vi "DEMO_02_READ_VOLT_S.vi"() -> ()   [LabVIEW 2018]
uses:
  <vilib>/Instr/_visa.llb/VISA Configure Serial Port (Instr).vi
panel:
  out "输出变量":dbl
  in  "打开串口":bool
  in  "通道选择":enum16{"一路", "二路", "三路"}(ring)
  in  "开闭环":u16(ring) items=["  开环", "  闭环"]
  in  "上位机控制":bool
  in  "读取数据":bool
  in  "VISA资源名称":refnum<visa-resource-name>="COM1"
  in  "波特率":u32(ring)=9600 items=["75"=75, "110"=110, "134"=134, "150"=150, "300"=300, "600"=600, "1200"=1200, "1800"=1800, "2400"=2400, "4800"=4800, "7200"=7200, "9600"=9600, "14400"=14400, "19200"=19200, "28800"=28800, "38400"=38400, "56000"=56000, "57600"=57600, "115200"=115200, "128000"=128000, "230400"=230400]
  in  "奇偶":enum16{"None", "Odd", "Even", "Mark", "Space"}(ring) caption="校验"
  # "发送数据以及读取开闭环数据"
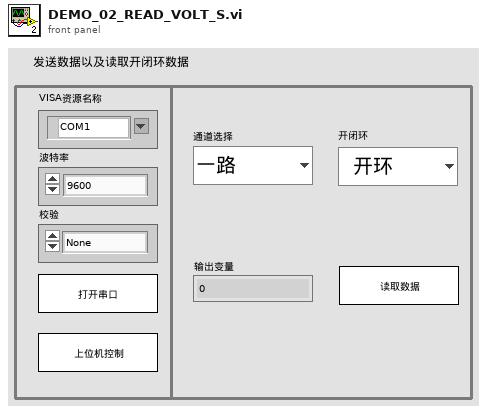
[diagram p1: front panel]
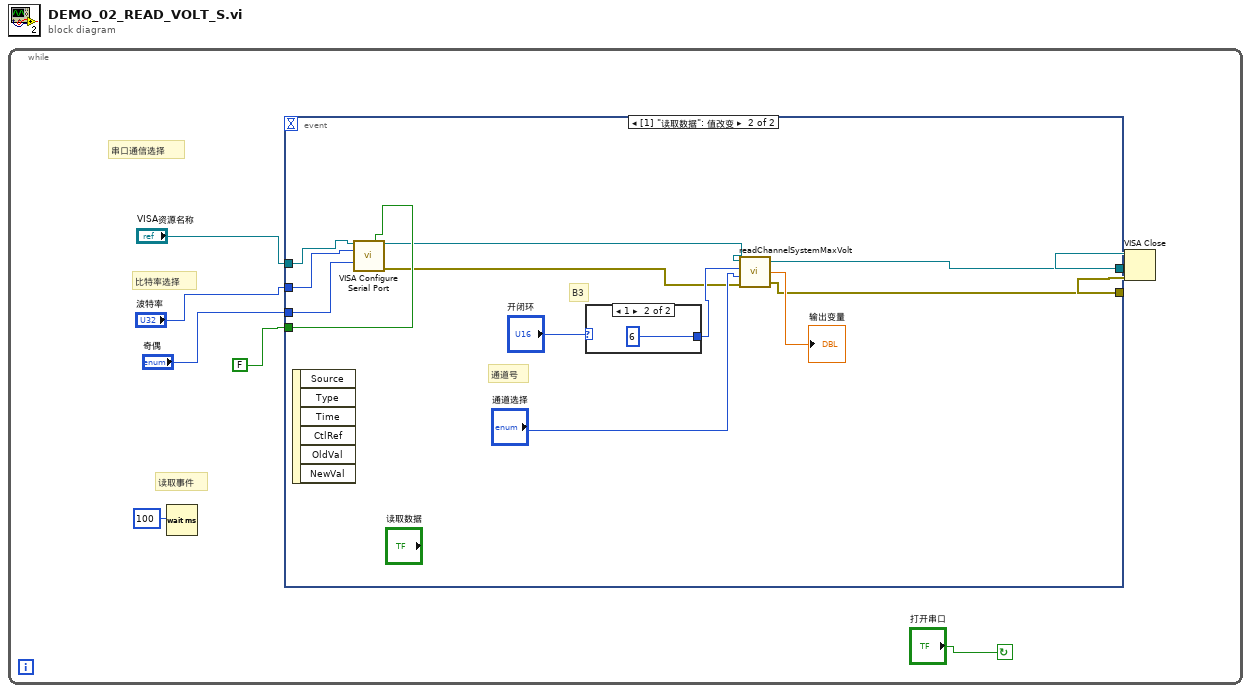
[diagram p0: block diagram]
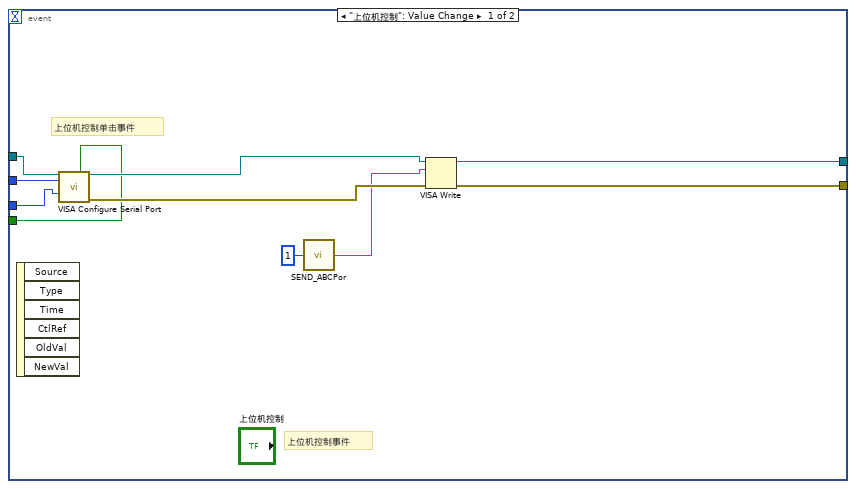
[diagram p2: hidden frame]
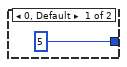
[diagram p3: hidden frame]
diagram:
  n1 = while {
    stop <- "打开串口" continue-if-true
    # "读取事件"
    # "比特率选择"
    # "串口通信选择"
    n2 = Wait (ms)(milliseconds to wait=100) -> ()  [unwired: 1 out]
    n3 = event shown="[1] \"读取数据\": 值改变" {
      selector: _ -> [_ _]
      dyn-events: _ -> [_ _]
      timeout: _ -> [_ _]
      tunnel: "VISA资源名称" -> [w18 w30]
      tunnel: "波特率" -> [w17 w29]
      tunnel: "奇偶" -> [w16 w28]
      tunnel: [w13 w20] -> w6
      tunnel: [w12 w19] -> w5
      tunnel: FALSE -> [w11 w27]
      event "上位机控制": Value Change {
        # "上位机控制事件"
        # "上位机控制单击事件"
        n4 = event-data() -> ()  [unwired: 1 in, 6 out]
        n5 = call-poly "VISA Configure Serial Port"("VISA resource name"=w18, "Enable Termination\nChar (T)"=w11, "baud rate (9600)"=w17, "parity (0:none)"=w16) -> ("VISA resource name out"=w15:refnum<visa-resource-name>, "error out"=w14:errorcluster)  [unwired: 10 in]
        n6 = call "SEND_ABCPor.vi"("设备地址 1 开始"=1) -> ("输出字符串"=w9:string)
        n7 = VISA Write(VISA resource name=w15, write buffer=w9, error in (no error)=w14) -> (VISA resource name out=w13:refnum<visa-resource-name>, error out=w12:errorcluster)  [unwired: 1 out]
      }
      event "读取数据": Value Change {
        # "通道号"
        # "B3"
        n8 = event-data() -> ()  [unwired: 1 in, 6 out]
        n9 = call-poly "VISA Configure Serial Port"("VISA resource name"=w30, "Enable Termination\nChar (T)"=w27, "baud rate (9600)"=w29, "parity (0:none)"=w28) -> ("VISA resource name out"=w22:refnum<visa-resource-name>, "error out"=w21:errorcluster)  [unwired: 10 in]
        n10 = case shown="1" "开闭环" {
          tunnel: [5 6] -> w24
          frame 0, Default {
          }
          frame 1 {
          }
        }
        n11 = call "readChannelSystemMaxVolt.vi"("error out 2"=w21, "通道号"="通道选择", "B3"=w24, "VISA resource name out 2"=w22) -> ("error out"=w19:errorcluster, "输出变量"=→"输出变量":dbl, "VISA resource name out"=w20:refnum<visa-resource-name>)
      }
    }
    n12 = VISA Close(VISA resource name=w6, error in (no error)=w5) -> ()  [unwired: 1 out]
  }
